vi "TurnCrank.vi"(8 "error in (no error)":errorcluster, 11 "GumballMachine in":refnum<class "GumballMachine.lvclass">) -> (0 "error out":errorcluster, 2 "ProcessMessage":string, 3 "GumballMachine out":refnum<class "GumballMachine.lvclass">)   [LabVIEW 2013, in "GumballMachine.lvclass"]
uses:
  GumballMachine.lvclass
  GumballMachine.lvclass/GumballMachine.ctl
  State.lvclass/State.lvclass
  StateMark.ctl
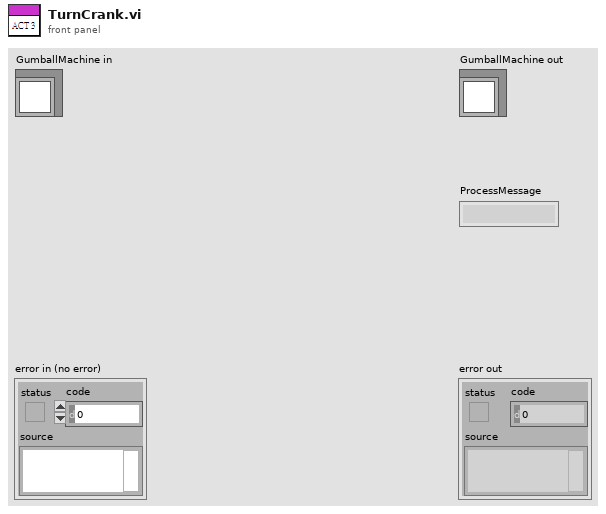
[diagram p1: front panel]
types:
  T1 = typedef "StateMark.ctl" = enum16{"沒有硬幣", "有硬幣", "賣出糖果", "糖果賣完", "NoChange"}
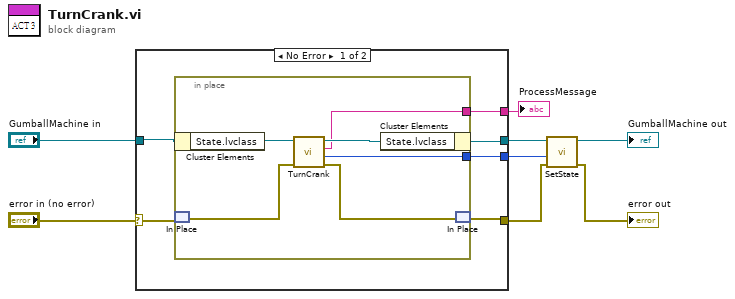
[diagram p0: block diagram]
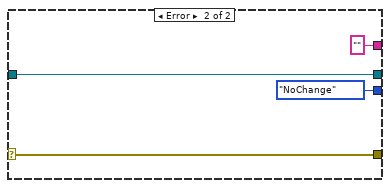
[diagram p2: hidden frame]
diagram:
  n1 = case shown="No Error" "error in (no error)" {
    selector: "error in (no error)" -> [w13 w24]
    tunnel: [w12 w24] -> w3
    tunnel: [w9 w23] -> w5
    tunnel: "GumballMachine in" -> [w14 w23]
    tunnel: [w11 StateMark."NoChange" ("NextState")] -> w4
    tunnel: [w10 "" ("ProcessMessage")] -> w6
    frame No Error {
      n2 = in-place {
        in-place-border: [w16] -> w11
        in-place-border: [w15] -> w10
        n3 = in-place-cluster #1(w14) -> ("State.lvclass"=w20:refnum<class "State.lvclass">)
        n4 = in-place-match #2(w13) -> (w18:errorcluster)
        n5 = call-dynamic "TurnCrank.vi"("error in (no error)"=w18, "State in"=w20) -> ("error out"=w17:errorcluster, "NextState"=w16:T1, "ProcessMessage"=w15:string, "State out"=w19:refnum<class "State.lvclass">)  [unwired: 6 in]
        n6 = in-place-cluster #1("State.lvclass"=w19) -> (w9:refnum<class "GumballMachine.lvclass">)
        n7 = in-place-match #2(w17) -> (w12:errorcluster)
      }
    }
    frame Error {
    }
  }
  "ProcessMessage" <- w6
  n8 = call-dynamic "SetState.vi"("error in (no error)"=w3, "State"=w4, "GumballMachine in"=w5) -> ("error out"=→"error out":errorcluster, "GumballMachine out"=→"GumballMachine out":refnum<class "GumballMachine.lvclass">)  [unwired: 7 in]
